vi "Vector fun.vi"() -> ()   [LabVIEW 2024]
uses:
  subs/Vector_typedef.ctl
panel:
  in  "Add Vectors":bool
  in  "vectors":T1[](array[typedef])=[{"vector"={"length"=30.0, "angle"=45.0, "sense"=TRUE}, "color"=0, "offset"={"X origin"=0, "Y origin"=0}}, {"vector"={"length"=70.0, "angle"=10.0, "sense"=TRUE}, "color"=16722176, "offset"={"X origin"=36, "Y origin"=60}}, {"vector"={"length"=30.0, "angle"=-15.0, "sense"=TRUE}, "color"=46165, "offset"={"X origin"=58, "Y origin"=18}}] {"offset"."Y origin" scale=0.0..100.0; "offset"."X origin" scale=0.0..100.0; "vector"."length" format="%.1f"; "vector"."angle" format="%.1f"}
  out "2D Picture":picture
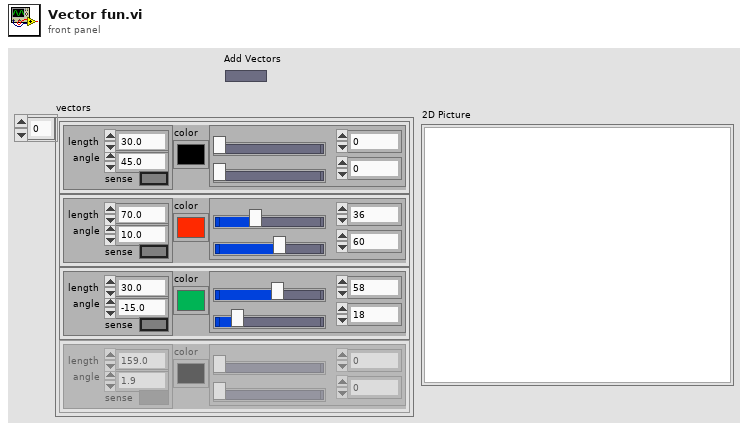
[diagram p1: front panel]
types:
  T1 = typedef "Vector_typedef.ctl" = cluster{"vector":cluster{"length":dbl, "angle":dbl, "sense":bool}, "color":u32, "offset":cluster{"X origin":i16, "Y origin":i16}}
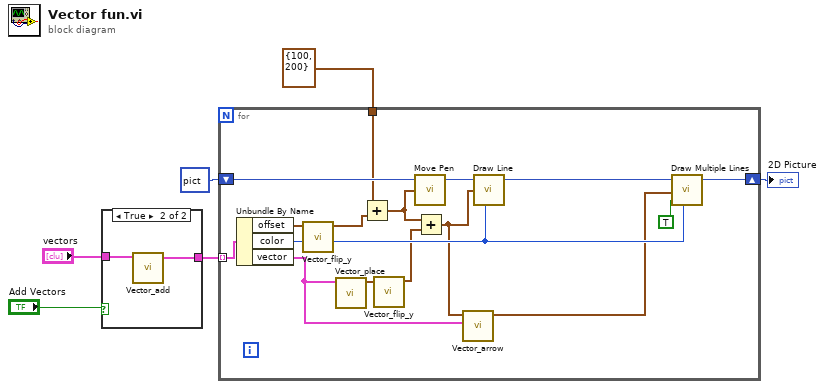
[diagram p0: block diagram]
diagram:
  n1 = case shown="True" "Add Vectors" {
    tunnel: "vectors" -> [w7 w9]
    tunnel: [w7 w8] -> w2
    frame False {
    }
    frame True {
      n2 = call "Vector_add.vi"("vectors"=w9) -> ("vectors"=w8:T1[])  [unwired: 10 in]
    }
  }
  n3 = for {
    tunnel: w2 -> [w24] mode=indexing
    shift-right: [w19] -> w6
    shift-left: picture data[5B] ("new picture") -> [w23]
    tunnel: cluster{"x":i16, "y":i16} {"x"=100, "y"=200} ("new position") -> [w22]
    n4 = Unbundle By Name(w24) -> ("offset"=w14:cluster{"X origin":i16, "Y origin":i16}, "color"=w18:u32, "vector"=w10:cluster{"length":dbl, "angle":dbl, "sense":bool})
    n5 = call "Vector_flip_y.vi"("x,y"=w14) -> ("x,-y"=w13:cluster{"X ":i16, "Y ":i16})  [unwired: 10 in]
    n6 = call "Vector_place.vi"("vector"=w10) -> ("x,y"=w12:cluster{dbl, dbl})  [unwired: 10 in]
    n7 = Add(x=w22, y=w13) -> (x+y=w21:cluster{i16, i16})
    n8 = call "Vector_flip_y.vi"("x,y"=w12) -> ("x,-y"=w11:cluster{"X ":i16, "Y ":i16})  [unwired: 10 in]
    n9 = call <vilib>:"Move Pen.vi"("new position"=w21, "picture"=w23) -> ("new picture"=w25:picture)  [unwired: 3 in]
    n10 = Add(x=w21, y=w11) -> (x+y=w16:cluster{i16, i16})
    n11 = call "Vector_arrow.vi"("vector"=w10, "tip"=w16) -> ("(x,y)"=w17:cluster{dbl, dbl}[])  [unwired: 9 in]
    n12 = call <vilib>:"Draw Line.vi"("picture"=w25, "end point"=w16, "color(black)"=w18) -> ("new picture"=w20:picture)  [unwired: 6 in]
    n13 = call <vilib>:"Draw Multiple Lines.vi"("picture"=w20, "line endpoints"=w17, "fill?(F)"=TRUE, "color(black)"=w18) -> ("new picture"=w19:picture)  [unwired: 5 in]
  }
  "2D Picture" <- w6
